vi "AudioTest.Save Waveform to CSV File.vi"(7 "Enable":bool, 9 "Root Name":string, 10 "Folder":path, 11 "Waveform":waveform(dbl)) -> (3 "Path":path)   [LabVIEW 2018]
uses:
  <vilib>/Waveform/WDTFileIO.llb/Export Waveform To Spreadsheet File.vi
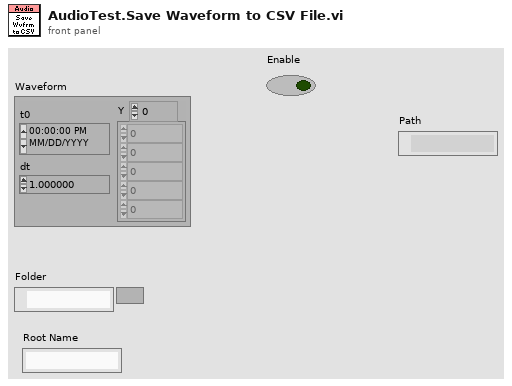
[diagram p1: front panel]
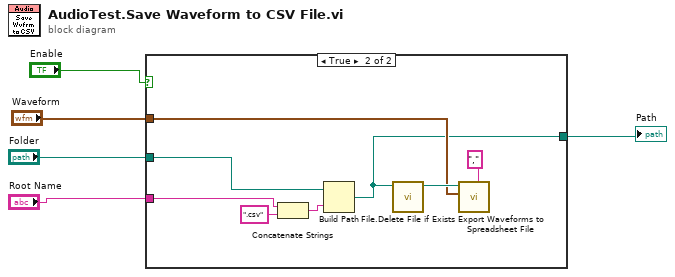
[diagram p0: block diagram]
diagram:
  n1 = case shown="True" "Enable" {
    tunnel: "Root Name" -> [_ w9]
    tunnel: "Folder" -> [_ w7]
    tunnel: "Waveform" -> [_ w8]
    tunnel: [_ w6] -> w1
    frame False {
    }
    frame True {
      n2 = Concatenate Strings(w9, ".csv" ("string")) -> (w13:string)
      n3 = Build Path(base path=w7, name or relative path=w13) -> (appended path=w6:path)
      n4 = call "File.Delete File if Exists.vi"("Path"=w6) -> ("Path Out"=w10:path)  [unwired: 9 in, 1 out]
      n5 = call-poly <vilib>:"Export Waveforms to Spreadsheet File.vi"("delimiter (Tab)"=",", "waveform"=w8, "file path (dialog if empty)"=w10) -> ()  [unwired: 7 in, 2 out]
    }
  }
  "Path" <- w1
